vi "Decode MSG of events.vi"(8 "error in (no error)":errorcluster, 11 "Domino Laser module Class in":refnum<class "Domino Laser module Class.lvclass">) -> (0 "error out":errorcluster, 1 "buffer ID":string, 2 "MSG ID":string, 3 "Domino Laser module Class out":refnum<class "Domino Laser module Class.lvclass">)   [LabVIEW 2015, in "Domino LM.lvlib" / "Domino Laser module Class.lvclass"]
uses:
  CTRLS/Domino Laser module Class.lvclass
  CTRLS/Domino Laser module Class.lvclass/Domino Laser module Class.ctl
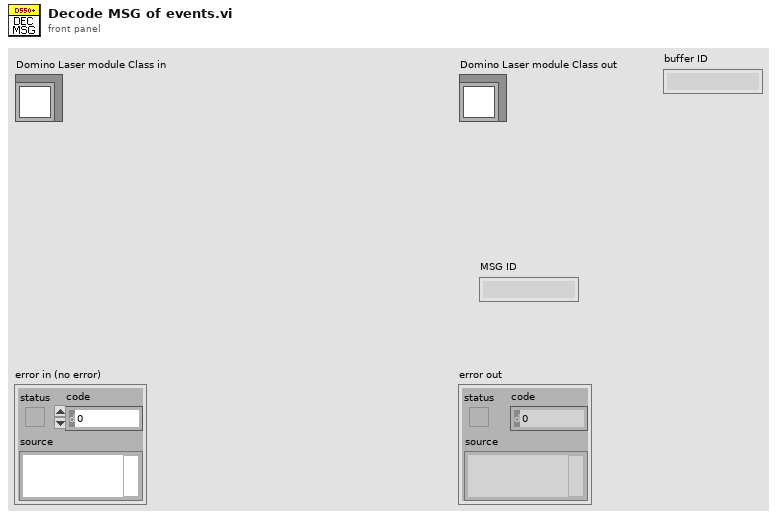
[diagram p1: front panel]
types:
  T1 = enum16{"Standard", "Buffered", "CRLF", "Immediate"}
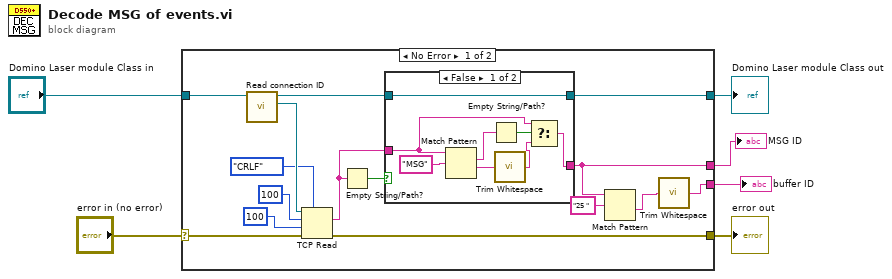
[diagram p0: block diagram]
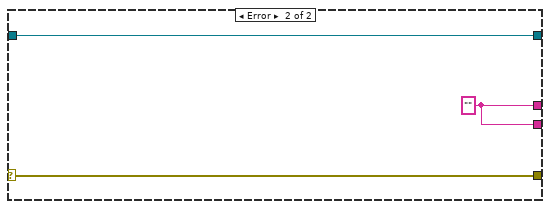
[diagram p3: hidden frame]
diagram:
  n1 = case shown="No Error" "error in (no error)" {
    selector: "error in (no error)" -> [w16 w34]
    tunnel: [w15 w34] -> w5
    tunnel: [w11 w33] -> w3
    tunnel: "Domino Laser module Class in" -> [w21 w33]
    tunnel: [w10 w32] -> w2
    tunnel: [w7 w32] -> w1
    frame No Error {
      n2 = call "Read connection ID.vi"("Domino Laser module Class in"=w21) -> ("connection ID"=w20:refnum<k5>, "Domino Laser module Class out"=w12:refnum<class "Domino Laser module Class.lvclass">)  [unwired: 8 in, 1 out]
      n3 = TCP Read(connection ID=w20, bytes to read=100, error in (no error)=w16, 7:T1."CRLF" ("mode (standard)"), 9:100 ("timeout ms (25000)")) -> (data out=w13:string, error out=w15:errorcluster)  [unwired: 1 out]
      n4 = Empty String/Path?(string/path=w13) -> (empty?=w14:bool)
      n5 = case shown="False" w14 {
        tunnel: w13 -> [w24 w31]
        tunnel: [w22 w31] -> w10
        tunnel: w12 -> [w27 w30]
        tunnel: [w27 w30] -> w11
        frame False {
          n6 = Match Pattern(string=w24, regular expression="MSG") -> (match substring=w25:string, after substring=w28:string)  [unwired: 1 in, 2 out]
          n7 = Empty String/Path?(string/path=w25) -> (empty?=w26:bool)
          n8 = call <vilib>:"Trim Whitespace.vi"("string"=w28) -> ("trimmed string"=w23:string)  [unwired: 1 in]
          n9 = Select(t=w24, s=w26, f=w23) -> (s? t:f=w22:string)
        }
        frame True {
        }
      }
      n10 = Match Pattern(string=w10, regular expression="25 ") -> (after substring=w8:string)  [unwired: 1 in, 3 out]
      n11 = call <vilib>:"Trim Whitespace.vi"("string"=w8) -> ("trimmed string"=w7:string)  [unwired: 1 in]
    }
    frame Error {
      w32 = "" ("trimmed string")
    }
  }
  "error out" <- w5
  "Domino Laser module Class out" <- w3
  "MSG ID" <- w2
  "buffer ID" <- w1
